vi "XY offset corrections.vi"   [LabVIEW 2019]
uses:
  <vilib>/Analysis/coordinate.llb/2D Cartesian Coordinate Rotation (Scalar).vi
  <vilib>/Analysis/baseanly.llb/Mean (DBL).vi
  <vilib>/Utility/file.llb/Write Delimited Spreadsheet (DBL).vi
  <vilib>/Analysis/NI_AALPro.lvlib
  <vilib>/Analysis/NI_AALBase.lvlib
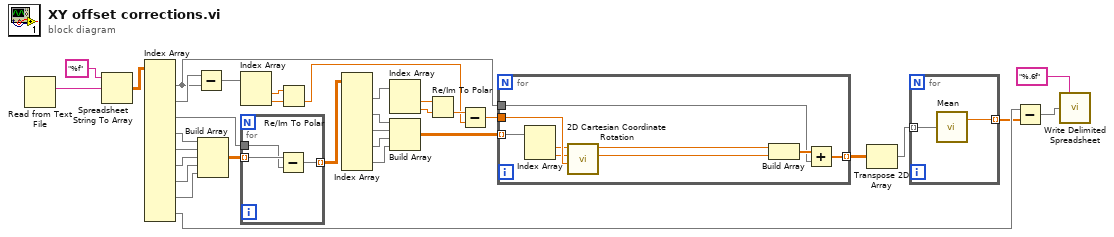
[diagram p0: block diagram]
diagram:
  n1 = Read from Text File() -> (text=w33:string)  [unwired: 4 in, 3 out]
  n2 = Spreadsheet String To Array(format string="%f", spreadsheet string=w33) -> (array=w31:dbl[][])  [unwired: 2 in]
  n3 = Index Array(array=w31) -> (element #1=w7:dbl[], element #2=w18:dbl[], element #3=w25:dbl[], element #4=w23:dbl[], element #5=w30:dbl[], element #6=w29:dbl[], element #7=w28:dbl[], element #8=w27:dbl[], element #9=w3:dbl[])  [unwired: 18 in]
  n4 = Subtract(x=w18, y=w7) -> (x-y=w17:dbl[])
  n5 = Build Array(w23, w30, w29, w28, w27) -> (w26:dbl[][])
  n6 = Index Array(array=w17) -> (element #1=w16:dbl, element #2=w15:dbl)  [unwired: 2 in]
  n7 = for {
    tunnel: w26 -> [w36] mode=indexing
    tunnel: w25 -> [w35]
    tunnel: [w34] -> w24 mode=indexing
    n8 = Subtract(x=w36, y=w35) -> (x-y=w34:dbl[])
  }
  n9 = Re/Im To Polar(2:w15, 3:w16) -> (0:w14:dbl)  [unwired: 1 out]
  n10 = Index Array(array=w24) -> (element #1=w22:dbl[], element #2=w12:dbl[], element #3=w11:dbl[], element #4=w10:dbl[], element #5=w9:dbl[])  [unwired: 10 in]
  n11 = Index Array(array=w22) -> (element #1=w21:dbl, element #2=w20:dbl)  [unwired: 2 in]
  n12 = Build Array(w12, w11, w10, w9) -> (w8:dbl[][])
  n13 = Re/Im To Polar(2:w20, 3:w21) -> (0:w19:dbl)  [unwired: 1 out]
  n14 = Subtract(x=w19, y=w14) -> (x-y=w13:dbl)
  n15 = for {
    tunnel: w13 -> [w45]
    tunnel: w8 -> [w42] mode=indexing
    tunnel: w7 -> [w38]
    tunnel: [w37] -> w5 mode=indexing
    n16 = Index Array(array=w42) -> (element #1=w44:dbl, element #2=w43:dbl)  [unwired: 2 in]
    n17 = call-poly <vilib>:"2D Cartesian Coordinate Rotation.vi"("theta"=w45, "y"=w43, "x"=w44) -> ("y out"=w40:dbl, "x out"=w41:dbl)  [unwired: 6 in, 1 out]
    n18 = Build Array(w41, w40) -> (w39:dbl[])
    n19 = Add(x=w39, y=w38) -> (x+y=w37:dbl[])
  }
  n20 = Transpose 2D Array(2D array=w5) -> (transposed array=w4:dbl[][])
  n21 = for {
    tunnel: w4 -> [w47] mode=indexing
    tunnel: [w46] -> w2 mode=indexing
    n22 = call-poly <vilib>:"Mean.vi"("X"=w47) -> ("mean"=w46:dbl)  [unwired: 1 out]
  }
  n23 = Subtract(x=w3, y=w2) -> (x-y=w1:dbl[])
  n24 = call-poly <vilib>:"Write Delimited Spreadsheet.vi"("format (%.3f)"="%.6f", "1D data"=w1) -> ()  [unwired: 12 in, 2 out]
